vi "soundstudio.vi"() -> ()   [LabVIEW 2018]
panel:
  out "?":dynamicdata(graph)
  in  "Lopass Cut-Off":dbl=100.0 caption="Lower Cut-Off"
  out "Waveform Graph":dynamicdata(graph)
  out "Lopass Filtered Signal":dynamicdata(graph) caption="Filtered Signal"
  out "Hipass Filtered Signal":dynamicdata(graph) caption="Filtered Signal"
  in  "Hipass Cut-Off":dbl=100.0 caption="Lower Cut-Off"
  in  "Speed factor":dbl
  in  "Loading path":path
  in  "Saving Path":path
  in  "Mode":T1(ring)
  in  "Record Duration (s)":dbl=1.0 caption="Duration (s)"
  # "Functionality requirement:\nThis vi should be able to: record audio, play back the audio, save to a file, play from a file, reverse the audio, speed up the audio, slow down the audio, and filter the audio (high pass, low pass)."
  # "_______________________________________________________________________________________________________"
  # "Recording Mode"
  # "(Time >0)"
  # "Saving Mode"
  # "`"
  # "Play from Selected File"
  # "(Use a different path than saving path \nbecause labVIEW will have issue handleing \nand allocating resource)"
  # "快进/慢进"
  # "< 1 for speed up\n>1 for slow down"
  # "High Pass Filter"
  # "Low Pass Filter"
  # "(Custome) Smoothing 低音"
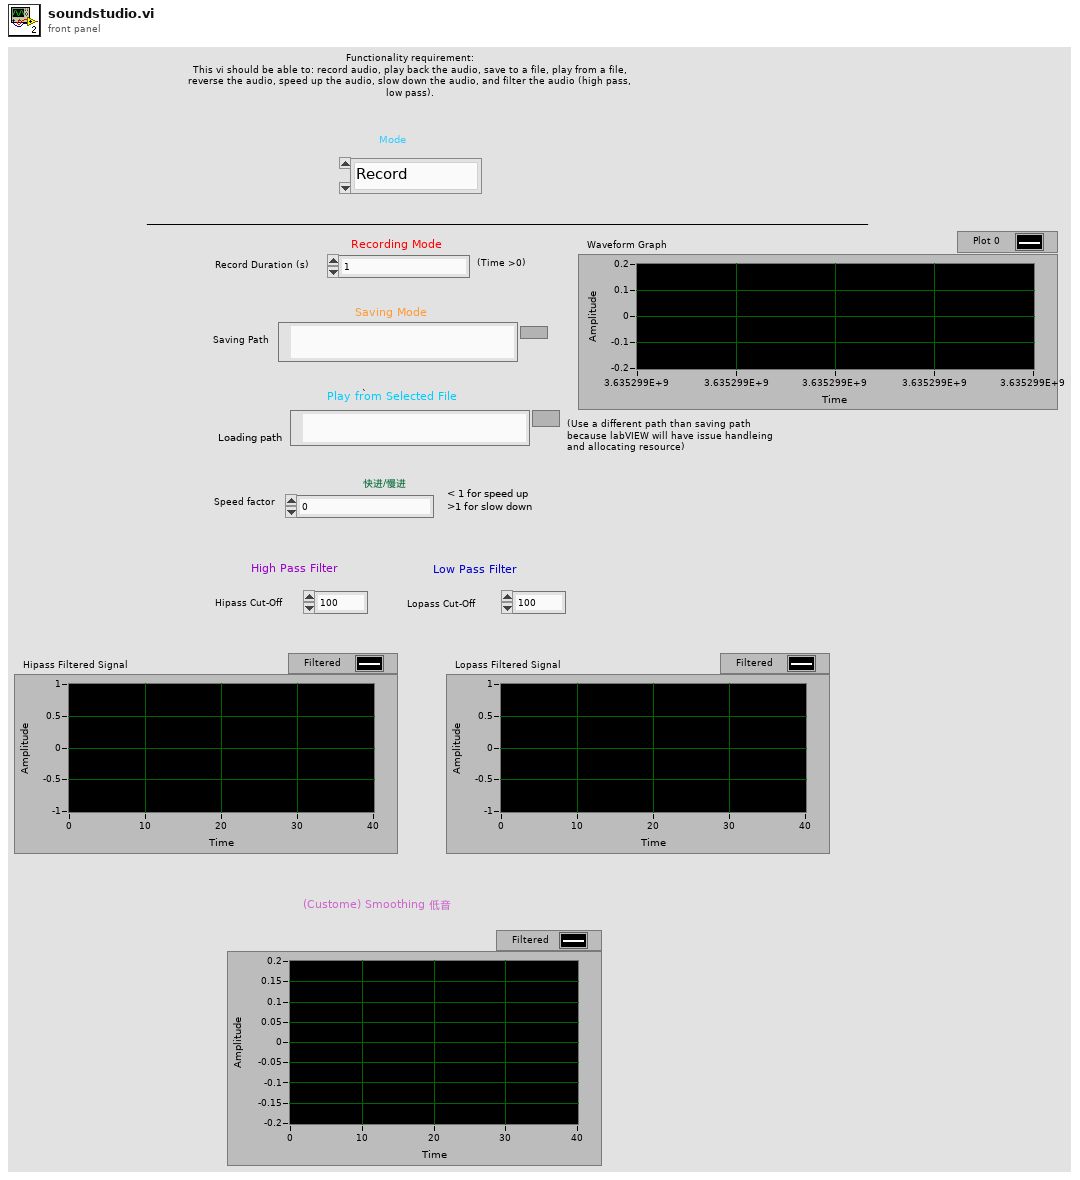
[diagram p1: front panel]
types:
  T1 = enum16{"Record", "Play back", "Save to file", "Play from file", "倒放", "快/慢 进", "High Pass Filter", "Low Pass Filter", "Custome (Volume)"}
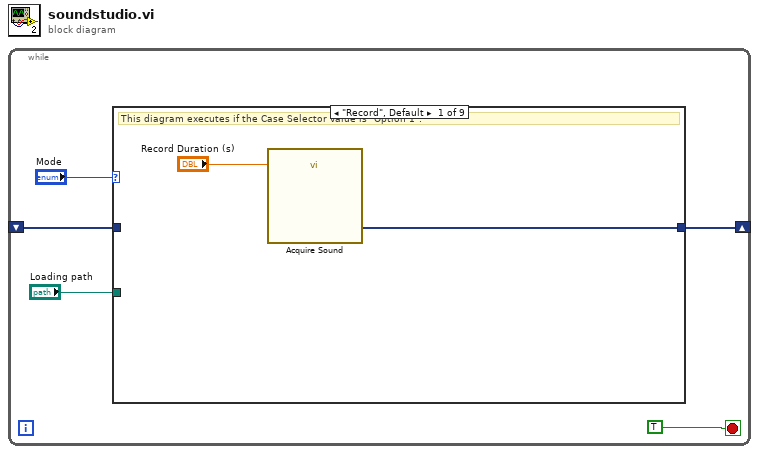
[diagram p0: block diagram]
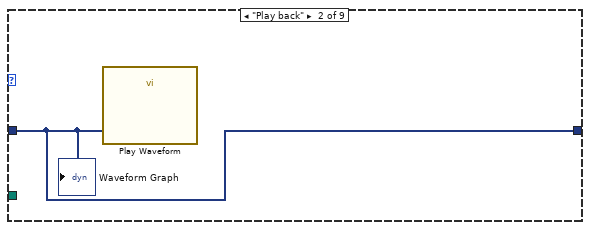
[diagram p2: hidden frame]
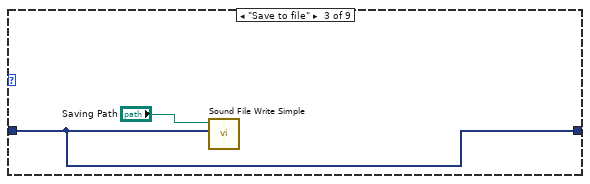
[diagram p3: hidden frame]
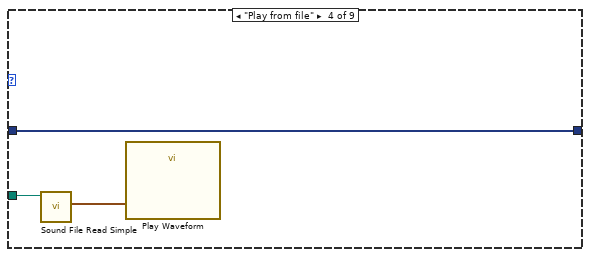
[diagram p4: hidden frame]
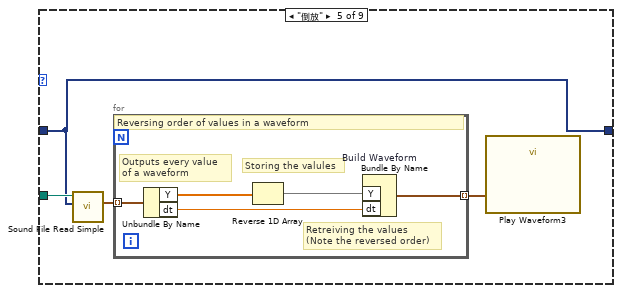
[diagram p5: hidden frame]
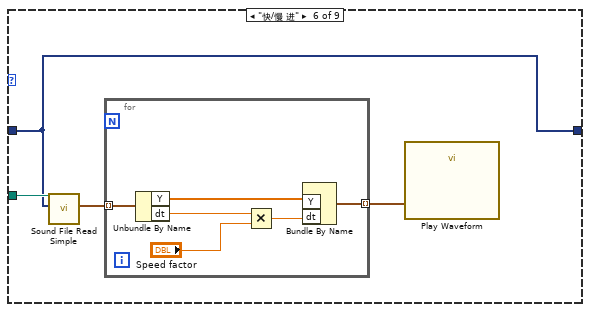
[diagram p6: hidden frame]
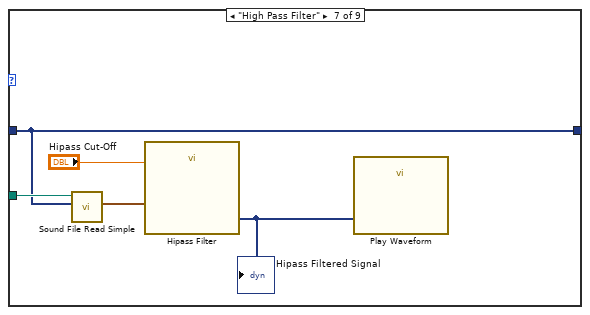
[diagram p7: hidden frame]
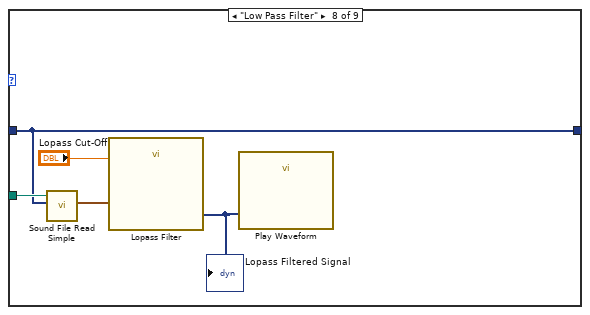
[diagram p8: hidden frame]
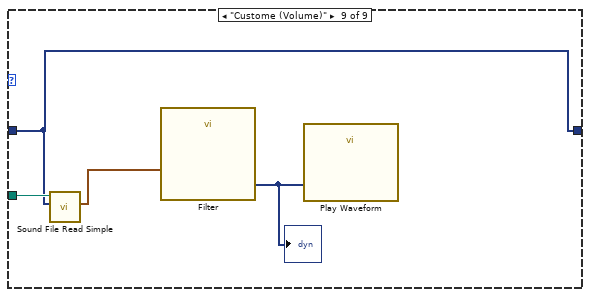
[diagram p9: hidden frame]
diagram:
  n1 = while {
    shift-right: [w5] -> _
    shift-left: _ -> [w3]
    stop <- TRUE stop-if-true
    n2 = case "Enum Case Structure" shown="\"Record\", Default" "Mode" {
      tunnel: [w6 w8 w9 w12 w14 w23 w35 w40 w45] -> w5
      tunnel: w3 -> [_ w8 w9 w12 w14 w23 w35 w40 w45]
      tunnel: "Loading path" -> [_ _ _ w11 w17 w26 w37 w42 w46]
      frame "Record", Default {
        # "This diagram executes if the Case Selector value is \"Option 1\"."
        n3 = call "Acquire Sound"("Duration (s)"="Record Duration (s)") -> ("Data"=w6:dynamicdata)  [unwired: 17 in, 1 out]
      }
      frame "Play back" {
        n4 = call "Play Waveform"("Data"=w8) -> ()  [unwired: 18 in, 1 out]
        "Waveform Graph" <- w8
      }
      frame "Save to file" {
        n5 = call <vilib>:"Sound File Write Simple.vi"("data"=w9, "path"="Saving Path") -> ()  [unwired: 8 in, 2 out]
      }
      frame "Play from file" {
        n6 = call <vilib>:"Sound File Read Simple.vi"("path"=w11) -> ("data"=w13:waveform(dbl)[])  [unwired: 7 in, 3 out]
        n7 = call "Play Waveform"("Data"=w13) -> ()  [unwired: 18 in, 1 out]
      }
      frame "倒放" {
        n8 = call <vilib>:"Sound File Read Simple.vi"("position mode"=w14, "path"=w17) -> ("data"=w16:waveform(dbl)[])  [unwired: 6 in, 3 out]
        n9 = for {
          tunnel: w16 -> [w22] mode=indexing
          tunnel: [w18] -> w15 mode=indexing
          # "Retreiving the values\n(Note the reversed order)"
          # "Storing the valules"
          # "Outputs every value \nof a waveform"
          # "Reversing order of values in a waveform"
          n10 = Unbundle By Name(w22) -> ("Y"=w21:dbl[], "dt"=w19:dbl)
          n11 = Reverse 1D Array(array=w21) -> (reversed array=w20:dbl[])
          n12 = Bundle By Name "Build Waveform"("Y"=w20, "dt"=w19) -> (w18:waveform(dbl))  [unwired: 1 in]
        }
        n13 = call "Play Waveform3"("Data"=w15) -> ()  [unwired: 18 in, 1 out]
      }
      frame "快/慢 进" {
        n14 = call <vilib>:"Sound File Read Simple.vi"("position mode"=w23, "path"=w26) -> ("data"=w25:waveform(dbl)[])  [unwired: 6 in, 3 out]
        n15 = for {
          tunnel: w25 -> [w32] mode=indexing
          tunnel: [w27] -> w24 mode=indexing
          n16 = Unbundle By Name ("Get Waveform Components")(w32) -> ("Y"=w28:dbl[], "dt"=w30:dbl)
          n17 = Multiply(x=w30, y="Speed factor") -> (x*y=w29:dbl)
          n18 = Bundle By Name ("Build Waveform")("Y"=w28, "dt"=w29) -> (w27:waveform(dbl))  [unwired: 1 in]
        }
        n19 = call "Play Waveform"("Data"=w24) -> ()  [unwired: 18 in, 1 out]
      }
      frame "High Pass Filter" {
        n20 = call <vilib>:"Sound File Read Simple.vi"("position mode"=w35, "path"=w37) -> ("data"=w36:waveform(dbl)[])  [unwired: 6 in, 3 out]
        n21 = call "Hipass Filter"("Lower Cut-Off"="Hipass Cut-Off", "Signal"=w36) -> ("Filtered Signal"=w33:dynamicdata)  [unwired: 8 in, 1 out]
        "Hipass Filtered Signal" <- w33
        n22 = call "Play Waveform"("Data"=w33) -> ()  [unwired: 18 in, 1 out]
      }
      frame "Low Pass Filter" {
        n23 = call <vilib>:"Sound File Read Simple.vi"("position mode"=w40, "path"=w42) -> ("data"=w41:waveform(dbl)[])  [unwired: 6 in, 3 out]
        n24 = call "Lopass Filter"("Lower Cut-Off"="Lopass Cut-Off", "Signal"=w41) -> ("Filtered Signal"=w39:dynamicdata)  [unwired: 8 in, 1 out]
        "Lopass Filtered Signal" <- w39
        n25 = call "Play Waveform"("Data"=w39) -> ()  [unwired: 18 in, 1 out]
      }
      frame "Custome (Volume)" {
        n26 = call <vilib>:"Sound File Read Simple.vi"("position mode"=w45, "path"=w46) -> ("data"=w44:waveform(dbl)[])  [unwired: 6 in, 3 out]
        n27 = call "Filter"("Signal"=w44) -> ("Filtered Signal"=w43:dynamicdata)  [unwired: 9 in, 1 out]
        "?" <- w43
        n28 = call "Play Waveform"("Data"=w43) -> ()  [unwired: 18 in, 1 out]
      }
    }
  }
